vi "VG-set_plot_names.vi"(11 "appended array":refnum<vi>[](array[refnum])) -> ()   [LabVIEW 2020, in "VG-VNA_GUI.lvlib" / "VG-VNA_GUI.lvclass"]
uses:
  VG-VNA_GUI.lvclass
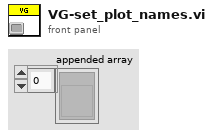
[diagram p1: front panel]
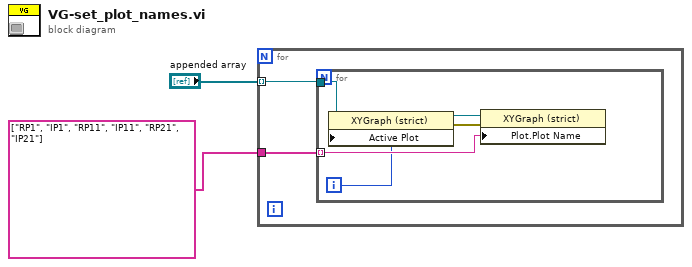
[diagram p0: block diagram]
diagram:
  n1 = for {
    tunnel: "appended array" -> [w4] mode=indexing
    tunnel: string[] ["RP1", "IP1", "RP11", "IP11", "RP21", "IP21"] -> [w3]
    n2 = for {
      tunnel: w4 -> [w9]
      tunnel: w3 -> [w6] mode=indexing
      i -> [w5]
      n3 = property class="XYGraph (strict)"(reference=w9, "Active Plot"=w5) -> (reference out=w8:refnum<vi>, error out=w7:errorcluster)  [unwired: 1 in]
      n4 = property class="XYGraph (strict)"(reference=w8, error in=w7, "Plot.Plot Name"=w6) -> ()  [unwired: 2 out]
    }
  }
